vi "Power Fit.vi"(9 "parameter bounds":T1, 10 "X":dbl[](array[numeric]), 11 "Y":dbl[](array[numeric])) -> (2 "Power Model":dbl[](array[numeric]), 3 "Fit Verification":cluster{dbl[], "Best Power Fit":dbl[]}[](array[cluster]))   [LabVIEW 2014, in "AvaSpec.lvlib" / "AvaSpec Logging.lvlib"]
uses:
  AvaSpec Logging.lvlib
  <vilib>/Analysis/NI_AALPro.lvlib
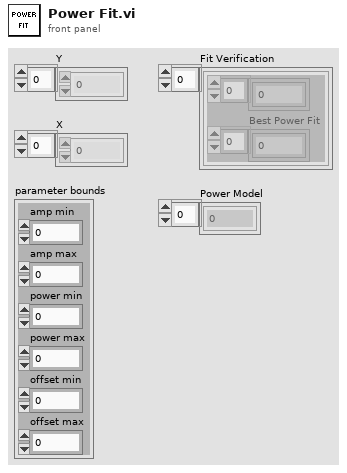
[diagram p1: front panel]
types:
  T1 = cluster{"amp min":dbl, "amp max":dbl, "power min":dbl, "power max":dbl, "offset min":dbl, "offset max":dbl}
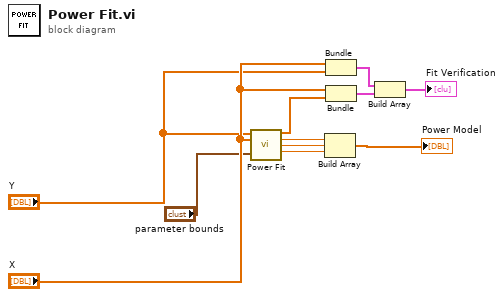
[diagram p0: block diagram]
diagram:
  n1 = call <vilib>:"Power Fit.vi"("Y"="Y", "X"="X", "parameter bounds"="parameter bounds") -> ("Best Power Fit"=w6:dbl[], "amplitude"=w1:dbl, "power"=w2:dbl, "offset"=w3:dbl)  [unwired: 7 in, 2 out]
  n2 = Build Array(w1, w2, w3) -> (→"Power Model":dbl[])
  n3 = Bundle("X"="X", "Y"="Y") -> (w7:cluster{"X":dbl[], "Y":dbl[]})  [unwired: 1 in]
  n4 = Bundle("X"="X", "Best Power Fit"=w6) -> (w8:cluster{"X":dbl[], "Best Power Fit":dbl[]})  [unwired: 1 in]
  n5 = Build Array(w7, w8) -> (→"Fit Verification":cluster{"X":dbl[], "Best Power Fit":dbl[]}[])
